vi "zad2.vi"() -> ()   [LabVIEW 2017]
uses:
  <vilib>/sound2/lvsound2.llb/Sound Data Format.ctl
  <vilib>/sound2/lvsound2.llb/Sampling Mode.ctl
  <vilib>/sound2/lvsound2.llb/Sound File Write Open.vi
  <vilib>/sound2/lvsound2.llb/Sound Input Read (DBL).vi
  <vilib>/sound2/lvsound2.llb/Sound File Write (DBL).vi
panel:
  in  "path":path
  out "Waveform Graph":waveform(dbl)[](graph)
  in  "stop":bool
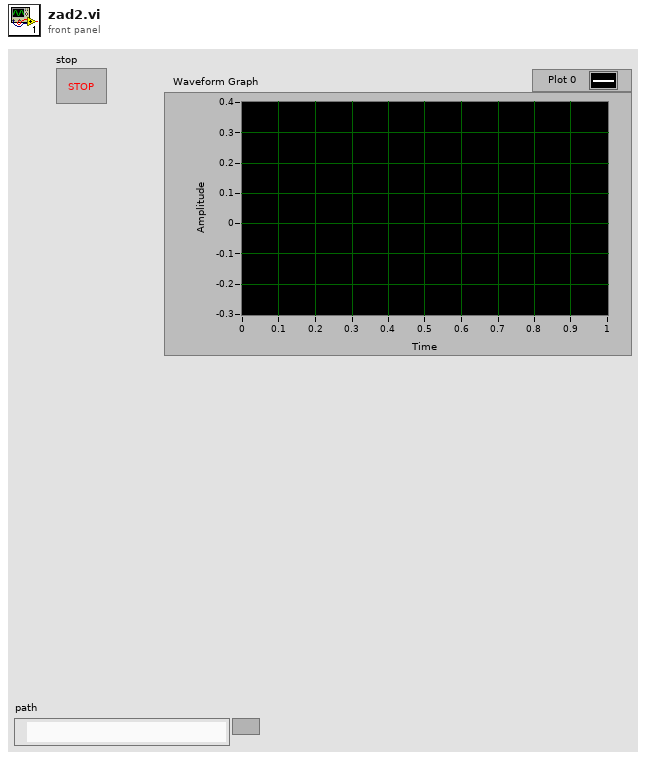
[diagram p1: front panel]
types:
  T1 = typedef "Sampling Mode.ctl" = i32
  T2 = typedef "Sound Data Format.ctl" = cluster{"sample rate (S/s)":dbl, "number of channels":i32, "bits per sample":i32}
  T3 = typedef "Sound File Refnum.ctl" = refnum<file>
  T4 = typedef "Sound Input Task ID.ctl" = u32
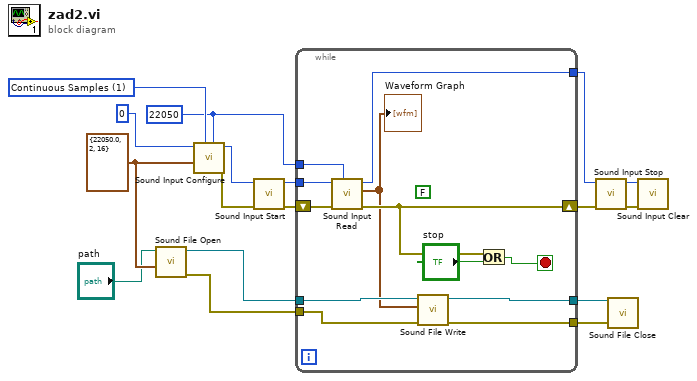
[diagram p0: block diagram]
diagram:
  w10 = T1 1 items=["Finite Samples", "Continuous Samples"] ("sample mode")
  w6 = T2 {"sample rate (S/s)"=22050.0, "number of channels"=2, "bits per sample"=16} ("sound format")
  w7 = 22050 ("number of samples/ch")
  n1 = call-poly <vilib>:"Sound File Open.vi"("sound format"=w6, "path"="path") -> ("error out"=w2:errorcluster, "sound file refnum"=w4:T3)  [unwired: 8 in]
  n2 = call <vilib>:"Sound Input Configure.vi"("number of samples/ch"=w7, "sample mode"=w10, "sound format"=w6, "device ID"=u32 0) -> ("error out"=w16:errorcluster, "task ID"=w12:T4)  [unwired: 6 in]
  n3 = call <vilib>:"Sound Input Start.vi"("error in (no error)"=w16, "task ID"=w12) -> ("error out"=w15:errorcluster, "task ID out"=w11:T4)  [unwired: 8 in]
  n4 = while {
    tunnel: w11 -> [w28]
    tunnel: w7 -> [w27]
    shift-right: [w25] -> w14
    shift-left: w15 -> [w29]
    tunnel: [w23] -> w9
    tunnel: w4 -> [w22]
    tunnel: [w21] -> w3
    tunnel: w2 -> [w20]
    tunnel: [w19] -> w1
    stop <- w24 stop-if-true
    (unwired) FALSE ("dB On (T)")
    n5 = call-poly <vilib>:"Sound Input Read.vi"("number of samples/ch"=w27, "error in (no error)"=w29, "task ID"=w28) -> ("error out"=w25:errorcluster, "data"=w18:waveform(dbl)[], "task ID out"=w23:T4)  [unwired: 6 in]
    "Waveform Graph" <- w18
    n6 = call-poly <vilib>:"Sound File Write.vi"("error in (no error)"=w20, "data"=w18, "sound file refnum"=w22) -> ("error out"=w19:errorcluster, "sound file refnum out"=w21:T3)  [unwired: 7 in]
    n7 = Or(x=w25, y="stop") -> (x .or. y?=w24:bool)
  }
  n8 = call <vilib>:"Sound Input Stop.vi"("error in (no error)"=w14, "task ID"=w9) -> ("error out"=w13:errorcluster, "task ID out"=w8:T4)  [unwired: 8 in]
  n9 = call <vilib>:"Sound File Close.vi"("error in (no error)"=w1, "sound file refnum"=w3) -> ()  [unwired: 9 in, 1 out]
  n10 = call <vilib>:"Sound Input Clear.vi"("error in (no error)"=w13, "task ID"=w8) -> ()  [unwired: 9 in, 1 out]
